vi "initialize.vi"(0 "heat_board_control in 2":refnum<class "heat_board_control.lvclass">, 5 "input channel":tag, 7 "PID":cluster{"P":dbl, "I":dbl, "D":dbl}, 9 "output channel":refnum<k21>, 11 "error in (no error)":errorcluster, 12 "sampling info":cluster{"Fs":dbl, "#s":dbl}={"Fs"=5000.0, "#s"=1000.0} {"Fs" format="%.2p"}, 13 "setpoint":path) -> (4 "heat_board_control out 2":refnum<class "heat_board_control.lvclass">, 15 "error out":errorcluster)   [LabVIEW 2015, in "heat_board_control.lvclass"]
uses:
  heat_board_control.lvclass
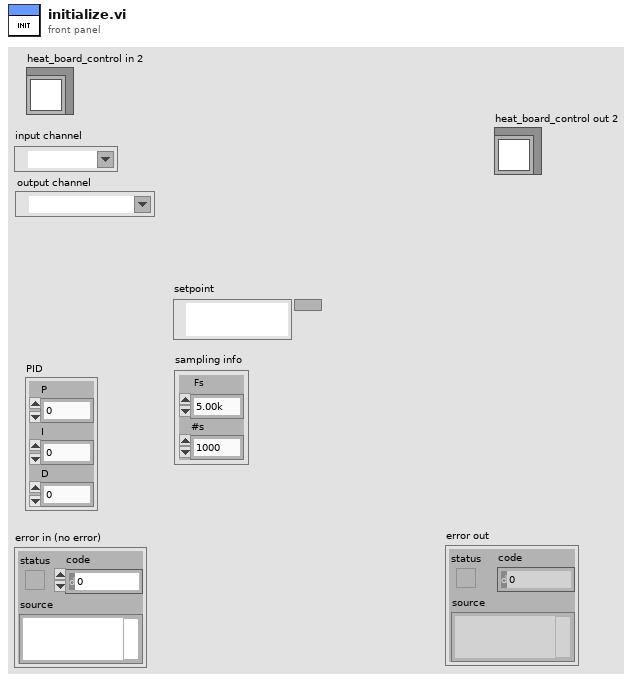
[diagram p1: front panel]
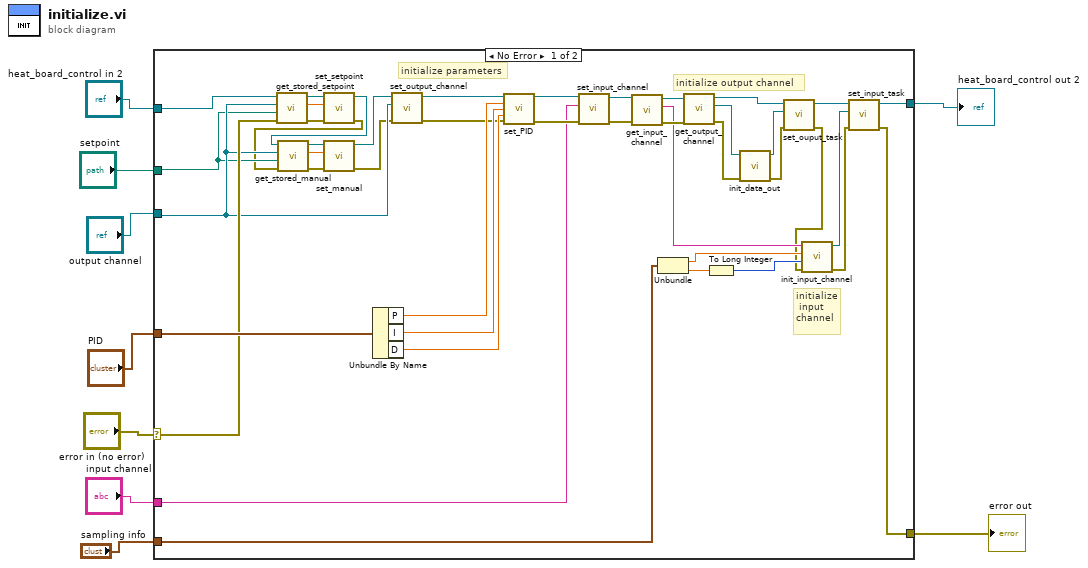
[diagram p0: block diagram]
diagram:
  n1 = case shown="No Error" "error in (no error)" {
    selector: "error in (no error)" -> [w34 w54]
    tunnel: [w22 w54] -> w8
    tunnel: [w26 w53] -> w6
    tunnel: "heat_board_control in 2" -> [w37 w53]
    tunnel: "output channel" -> [w18 _]
    tunnel: "PID" -> [w47 _]
    tunnel: "input channel" -> [w44 _]
    tunnel: "setpoint" -> [w17 _]
    tunnel: "sampling info" -> [w30 _]
    frame No Error {
      # "initialize parameters"
      # "initialize\n input \nchannel"
      # "initialize output channel"
      n2 = call-dynamic "get_stored_setpoint.vi"("error in (no error)"=w34, "connection information"=w17, "output channel"=w18, "heat_board_control in"=w37) -> ("error out"=w35:errorcluster, "setpoint"=w36:dbl, "heat_board_control out"=w38:refnum<class "heat_board_control.lvclass">)  [unwired: 5 in]
      n3 = call-dynamic "set_setpoint.vi"("error in (no error)"=w35, "setpoint"=w36, "heat_board_control in"=w38) -> ("error out"=w16:errorcluster, "heat_board_control out"=w15:refnum<class "heat_board_control.lvclass">)  [unwired: 7 in]
      n4 = call-dynamic "get_stored_manual.vi"("error in (no error)"=w16, "connection information"=w17, "output channel"=w18, "heat_board_control in"=w15) -> ("error out"=w12:errorcluster, "manual laser"=w19:dbl, "heat_board_control out"=w20:refnum<class "heat_board_control.lvclass">)  [unwired: 5 in]
      n5 = call-dynamic "set_manual.vi"("error in (no error)"=w12, "setpoint"=w19, "heat_board_control in"=w20) -> ("error out"=w14:errorcluster, "heat_board_control out"=w13:refnum<class "heat_board_control.lvclass">)  [unwired: 7 in]
      n6 = Unbundle By Name(w47) -> ("P"=w50:dbl, "I"=w51:dbl, "D"=w52:dbl)
      n7 = call-dynamic "set_output_channel.vi"("error in (no error)"=w14, "set output"=w18, "heat_board_control in"=w13) -> ("error out"=w10:errorcluster, "heat_board_control out"=w11:refnum<class "heat_board_control.lvclass">)  [unwired: 7 in]
      n8 = call-dynamic "set_PID.vi"("heat_board_control in"=w11, "P"=w50, "I"=w51, "D"=w52, "error in (no error)"=w10) -> ("heat_board_control out"=w46:refnum<class "heat_board_control.lvclass">, "error out"=w45:errorcluster)  [unwired: 9 in]
      n9 = call-dynamic "set_input_channel.vi"("error in (no error)"=w45, "input channel"=w44, "heat_board_control in"=w46) -> ("error out"=w41:errorcluster, "heat_board_control out"=w43:refnum<class "heat_board_control.lvclass">)  [unwired: 7 in]
      n10 = call-dynamic "get_input_channel.vi"("error in (no error)"=w41, "heat_board_control in"=w43) -> ("error out"=w40:errorcluster, "input channel"=w39:tag, "heat_board_control out"=w42:refnum<class "heat_board_control.lvclass">)  [unwired: 7 in]
      n11 = Unbundle(w30) -> ("Fs"=w32:dbl, "#s"=w33:dbl)
      n12 = call-dynamic "get_output_channel.vi"("error in (no error)"=w40, "heat_board_control in"=w42) -> ("error out"=w49:errorcluster, "physical channel"=w48:refnum<k21>, "heat_board_control out"=w28:refnum<class "heat_board_control.lvclass">)  [unwired: 7 in]
      n13 = To Long Integer(number=w33) -> (32bit integer=w31:i32)
      n14 = call "init_data_out.vi"("error in (no error)"=w49, "output channel"=w48) -> ("error out"=w24:errorcluster, "task out"=w29:refnum<k24>)  [unwired: 8 in]
      n15 = call-dynamic "set_ouput_task.vi"("error in (no error)"=w24, "output task in"=w29, "heat_board_control in"=w28) -> ("error out"=w21:errorcluster, "heat_board_control out"=w27:refnum<class "heat_board_control.lvclass">)  [unwired: 7 in]
      n16 = call "init_input_channel.vi"("error in (no error)"=w21, "samples per channel"=w31, "rate"=w32, "input channel"=w39) -> ("error out"=w23:errorcluster, "task out"=w25:refnum<k21>)  [unwired: 6 in]
      n17 = call-dynamic "set_input_task.vi"("error in (no error)"=w23, "input task out"=w25, "heat_board_control in"=w27) -> ("error out"=w22:errorcluster, "heat_board_control out"=w26:refnum<class "heat_board_control.lvclass">)  [unwired: 7 in]
    }
    frame Error {
    }
  }
  "error out" <- w8
  "heat_board_control out 2" <- w6
